vi "Program LCM.vi"(8 "error in (no error)":errorcluster, 11 "LCM Single-Up APP Programming in":refnum<class "LCM Single-Up APP Programming.lvclass">) -> (0 "error out":errorcluster, 2 "Success":bool, 3 "LCM Single-Up APP Programming out":refnum<class "LCM Single-Up APP Programming.lvclass">)   [LabVIEW 2015, in "LCM Single-Up APP Programming.lvclass"]
uses:
  LCM Single-Up APP Programming.lvclass
  Classes/Programmer/Segger Flasher ARM/Class/Segger Flasher ARM.lvclass
  Classes/Programmer/Programmer/Class/Programmer.lvclass
  Test Class/Test Class.lvclass
  Classes/Test Recipe/Class/Test Recipe.lvclass
  Classes/Application/Class/Application.lvclass
  <vilib>/Cree, Inc/Cree Test Framework/Classes/Base Objects/Base Class/Base Class/Base Class.lvclass
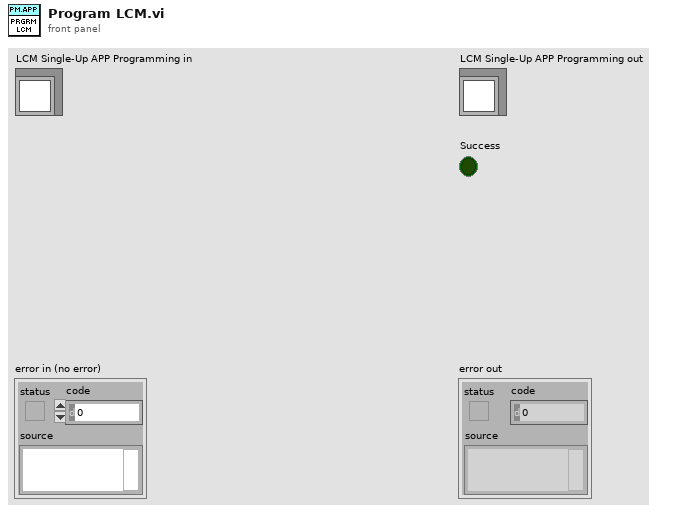
[diagram p1: front panel]
types:
  T1 = typedef "Application.lvlib/App Properties.lvclass/Class Properties -- Cluster.ctl" = cluster{"UUT Info":T2[], "Test Information":refnum<vi>, "Test Complete Event":refnum<user-event>, "Shop Floor System":refnum<class "Shop Floor System.lvclass">, "Gold Board":refnum<class "Golden Board.lvclass">, "Test Recipe":refnum<class "Test Recipe.lvclass">, "Instruments":refnum<class "Instrument.lvclass">[], "Mode":T3, "Test Results":cluster{"Pass":bool[], "Fail Codes":string[]}, "Station Config":refnum<class "Station Config.lvclass">}
  T2 = typedef "Application.lvlib/App Properties.lvclass/UUT Reference -- Cluster.ctl" = cluster{"Serial Number Reference":refnum<vi>, "Status Message Reference":refnum<vi>}
  T3 = typedef "Application.lvlib/Application.lvclass/Op Mode -- Enum.ctl" = u16
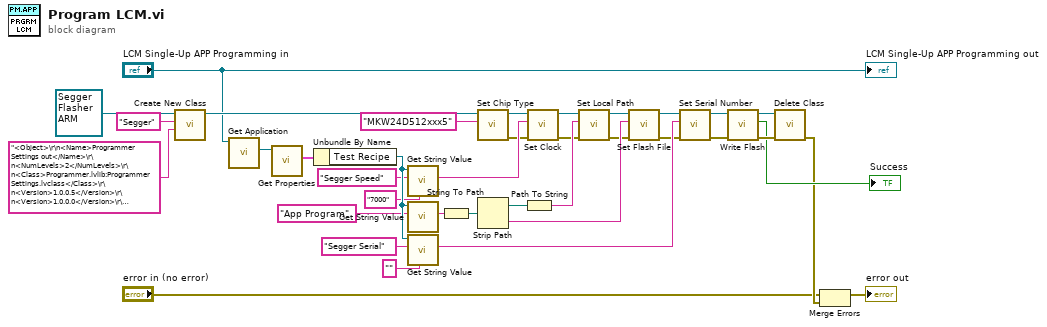
[diagram p0: block diagram]
diagram:
  n1 = call <vilib>:"Create New Class.vi"("Configuration"="<Object>\r\n<Name>Programmer Settings out</Name>\r\n<NumLevels>2</NumLevels>\r\n<Class>Programmer.lvlib:Programmer Settings.lvclass</Class>\r\n<Version>1.0.0.5</Version>\r\n<Version>1.0.0.0</Version>\r\n<Cluster>\r\n</Cluster>\r\n<Cluster>\r\n<Name>Programmer Settings.lvclass</Name>\r\n<NumElts>1</NumElts>\r\n<Cluster>\r\n<Name>Class Settings</Name>\r\n<NumElts>12</NumElts>\r\n<String>\r\n<Name>Local Path</Name>\r\n<Val>C:\\Programmer</Val>\r\n</String>\r\n<String>\r\n<Name>Network Path</Name>\r\n<Val>W:\\Programmer</Val>\r\n</String>\r\n<Boolean>\r\n<Name>Local Enable</Name>\r\n<Val>1</Val>\r\n</Boolean>\r\n<String>\r\n<Name>System Version</Name>\r\n<Val>v1.5</Val>\r\n</String>\r\n<String>\r\n<Name>Flash Hex File</Name>\r\n<Val></Val>\r\n</String>\r\n<String>\r\n<Name>Lockbits Hex File</Name>\r\n<Val></Val>\r\n</String>\r\n<String>\r\n<Name>Fuse Hex File</Name>\r\n<Val></Val>\r\n</String>\r\n<String>\r\n<Name>Revision</Name>\r\n<Val>1.05.207</Val>\r\n</String>\r\n<String>\r\n<Name>Chip Type</Name>\r\n<Val></Val>\r\n</String>\r\n<String>\r\n<Name>JTAG Serial Number</Name>\r\n<Val></Val>\r\n</String>\r\n<String>\r\n<Name>JTAG Clock</Name>\r\n<Val>6mhz</Val>\r\n</String>\r\n<I32>\r\n<Name>Number of Retries</Name>\r\n<Val>2</Val>\r\n</I32>\r\n</Cluster>\r\n</Cluster>\r\n</Object>\r\n" ("xml string"), "Name"="Segger", "Base Class in"=refnum<class "Segger Flasher ARM.lvclass"> refnum ("Segger Flasher ARM.lvlib:Segger Flasher ARM.lvclass")) -> ("Base Class out"=w33:refnum<class "Segger Flasher ARM.lvclass">)  [unwired: 7 in, 1 out]
  n2 = call "Get Application.vi"("Test Class in"="LCM Single-Up APP Programming in") -> ("Application.lvlib:Application.lvclass"=w25:refnum<class "Application.lvclass">)  [unwired: 9 in, 1 out]
  n3 = call "Get Properties.vi"("Acrobat Template in"=w25) -> ("Class Properties"=w23:T1)  [unwired: 8 in, 2 out]
  n4 = Unbundle By Name(w23) -> ("Test Recipe"=w24:refnum<class "Test Recipe.lvclass">)
  n5 = call "Get String Value.vi"("Default Value"="7000", "Name"="Segger Speed", "Test Recipe in"=w24) -> ("Value"=w28:string)  [unwired: 6 in, 2 out]
  n6 = call "Get String Value.vi"("Name"="App Program", "Test Recipe in"=w24) -> ("Value"=w26:string)  [unwired: 7 in, 2 out]
  n7 = call "Get String Value.vi"("Default Value"="", "Name"="Segger Serial", "Test Recipe in"=w24) -> ("Value"=w29:string)  [unwired: 6 in, 2 out]
  n8 = String To Path(string=w26) -> (path=w27:path)
  n9 = call "Set Chip Type.vi"("Chip Type"="MKW24D512xxx5", "Programmer in"=w33) -> ("error out"=w5:errorcluster, "Programmer out"=w13:refnum<class "Segger Flasher ARM.lvclass">)  [unwired: 8 in]
  n10 = Strip Path(path=w27) -> (stripped path=w14:path, name=w16:string)
  n11 = Path To String(path=w14) -> (string=w15:string)
  n12 = call "Set Clock.vi"("error in (no error)"=w5, "Clock Speed"=w28, "Programmer in"=w13) -> ("error out"=w6:errorcluster, "Programmer out"=w12:refnum<class "Segger Flasher ARM.lvclass">)  [unwired: 7 in]
  n13 = call "Set Local Path.vi"("error in (no error)"=w6, "Local Path"=w15, "Programmer in"=w12) -> ("error out"=w7:errorcluster, "Programmer out"=w11:refnum<class "Segger Flasher ARM.lvclass">)  [unwired: 7 in]
  n14 = call "Set Flash File.vi"("error in (no error)"=w7, "Flash File"=w16, "Programmer in"=w11) -> ("error out"=w8:errorcluster, "Programmer out"=w10:refnum<class "Segger Flasher ARM.lvclass">)  [unwired: 7 in]
  n15 = call "Set Serial Number.vi"("error in (no error)"=w8, "Serial Number"=w29, "Programmer in"=w10) -> ("error out"=w9:errorcluster, "Programmer out"=w17:refnum<class "Segger Flasher ARM.lvclass">)  [unwired: 7 in]
  n16 = call-dynamic "Write Flash.vi"("error in (no error)"=w9, "Acrobat Template in"=w17) -> ("error out"=w37:errorcluster, "Success"=→"Success":bool, "Acrobat Template out"=w34:refnum<class "Segger Flasher ARM.lvclass">)  [unwired: 6 in, 1 out]
  n17 = call <vilib>:"Delete Class.vi"("error in (no error)"=w37, "Base Class in"=w34) -> ("error out"=w35:errorcluster)  [unwired: 8 in, 1 out]
  n18 = Merge Errors("error in (no error)", w35) -> (→"error out":errorcluster)
  "LCM Single-Up APP Programming out" <- "LCM Single-Up APP Programming in"
